vi "报告生成子VI.vi"(5 "column width (1)":dbl=10.0 format="%#_13g", 6 "error in (no error)":errorcluster caption="错误输入（无错误）", 7 "产品编号":string, 8 "text data":string[][](array[string]) caption="文本数据", 9 "报告保存路径":path, 10 "标注后的图片路径":path, 11 "报告模板路径":path) -> (2 "报告存储路径":path, 3 "标注后的图片存储路径":path)   [LabVIEW 2018]
uses:
  <vilib>/Utility/NIReport.llb/HTML Report Image Alignment.ctl
  <vilib>/Utility/NIReport.llb/Report Type.ctl
  <vilib>/Utility/NIReport.llb/Append Report Text (str wrap).vi
  <vilib>/Utility/NIReport.llb/Append Text Table to Report (wrap).vi
  <vilib>/Utility/NIReport.llb/Append Image to Report (path wrap).vi
  <vilib>/Utility/NIReport.llb/NI_report.lvclass
  <vilib>/Utility/NIReport.llb/Word/NI_Word.lvclass
  <vilib>/Utility/NIReport.llb/NI_ReportGenerationCore.lvlib
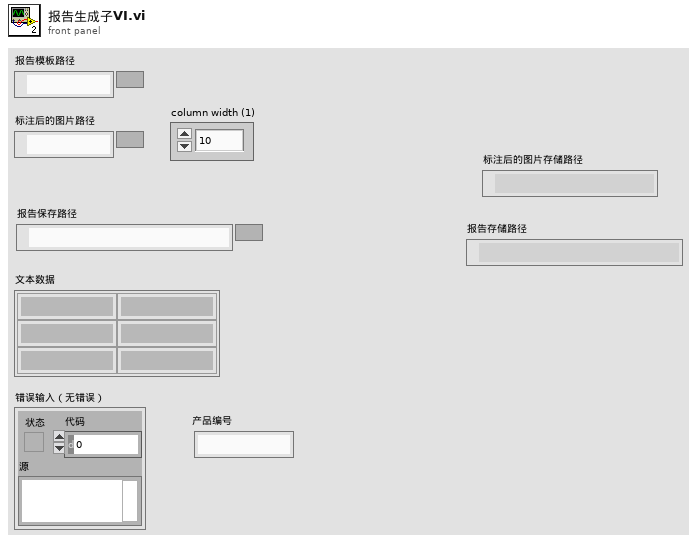
[diagram p1: front panel]
types:
  T1 = typedef "NI_ReportGenerationCore.lvlib/Report Type.ctl" = enum16{"HTML", "Word", "Excel"}
  T2 = cluster{"position (excel)":cluster{"row":i32, "column":i32}, "name (excel)":string, "bookmark (word)":string}
  T3 = typedef "NI_ReportGenerationCore.lvlib/HTML Report Image Alignment.ctl" = enum16{"(default)", "LEFT", "RIGHT", "TOP", "TEXTTOP", "MIDDLE", "ABSMIDDLE", "BASELINE", "BOTTOM", "ABSBOTTOM"}
  T4 = enum16{"maximized", "minimized", "normal", "no change"}
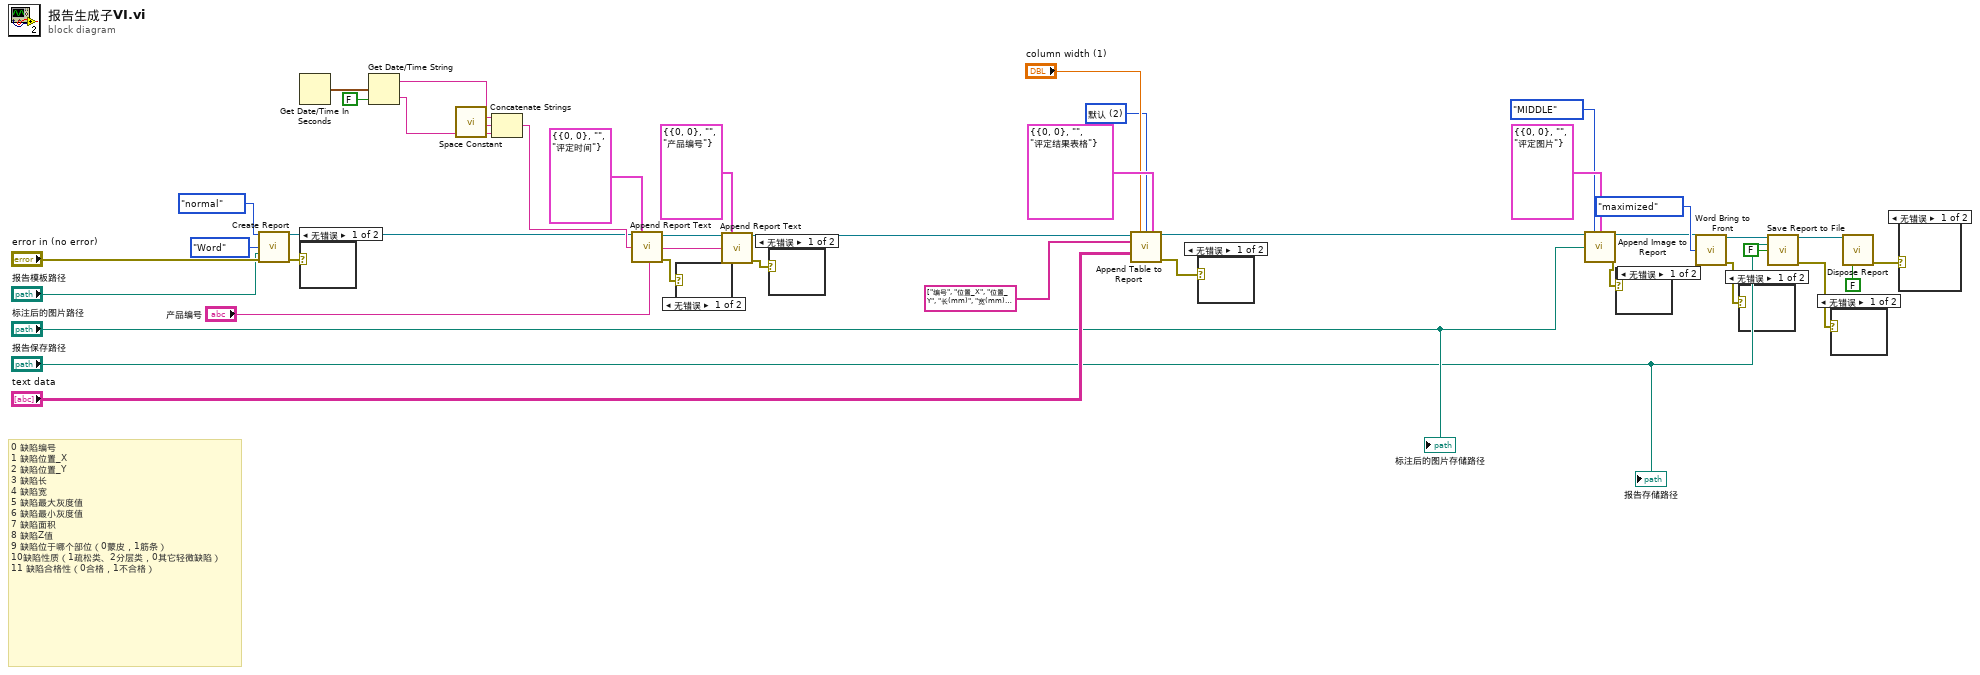
[diagram p0: block diagram]
diagram:
  w5 = u16 2 items=["US", "公制", "默认"] ("measurement system")
  # "0 缺陷编号\n1 缺陷位置_X\n2 缺陷位置_Y\n3 缺陷长\n4 缺陷宽\n5 缺陷最大灰度值\n6 缺陷最小灰度值\n7 缺陷面积\n8 缺陷Z值\n9 缺陷位于哪个部位（0蒙皮，1筋条）\n10缺陷性质（1疏松类、2分层类，0其它轻微缺陷）\n11 缺陷合格性（0合格，1不合格）"
  n1 = call <vilib>:"Create Report.vi"("window state (normal)"=T4."normal", "report type"=Report_Type."Word", "template (empty)"="报告模板路径", "error in (no error)"="error in (no error)") -> ("report out"=w1:refnum<class "NI_report.lvclass">, "error out"=w6:errorcluster)  [unwired: 10 in]
  n2 = Get Date/Time In Seconds() -> (seconds since 1Jan1904=w39:timestamp)
  n3 = case shown="无错误" w6 {
    frame No Error {
    }
    frame Error {
    }
  }
  n4 = Get Date/Time String(seconds (now)=w39, want seconds? (F)=FALSE ("需要秒？(F)")) -> (date string=w34:string, time string=w36:string)  [unwired: 1 in]
  n5 = call <vilib>:"Space Constant.vi"() -> ("String"=w33:string)
  n6 = Concatenate Strings(w34, w33, w36) -> (w35:string)
  n7 = call-poly <vilib>:"Append Report Text.vi"("report in"=w1, "MS Office parameters"=T2 {"position (excel)"={"row"=0, "column"=0}, "name (excel)"="", "bookmark (word)"="评定时间"}, "text"=w35) -> ("report out"=w26:refnum<class "NI_report.lvclass">, "error out"=w7:errorcluster)  [unwired: 9 in, 2 out]
  n8 = case shown="无错误" w7 {
    frame No Error {
    }
    frame Error {
    }
  }
  n9 = call-poly <vilib>:"Append Report Text.vi"("report in"=w26, "MS Office parameters"=T2 {"position (excel)"={"row"=0, "column"=0}, "name (excel)"="", "bookmark (word)"="产品编号"}, "text"="产品编号") -> ("report out"=w3:refnum<class "NI_report.lvclass">, "error out"=w4:errorcluster)  [unwired: 9 in, 2 out]
  n10 = case shown="无错误" w4 {
    frame No Error {
    }
    frame Error {
    }
  }
  n11 = call-poly <vilib>:"Append Table to Report.vi"("report in"=w3, "column width (1)"="column width (1)", "measurement system"=w5, "MS Office parameters"=T2 {"position (excel)"={"row"=0, "column"=0}, "name (excel)"="", "bookmark (word)"="评定结果表格"}, "column headers"=string[] ["编号", "位置_X", "位置_Y", "长(mm)", "宽(mm)", "最大灰度值", "最小灰度值", "面积(mm2)", "Z值(mm)", "部位", "类型", "合格性"], "text data"="text data") -> ("report out"=w2:refnum<class "NI_report.lvclass">, "error out"=w18:errorcluster)  [unwired: 6 in, 2 out]
  n12 = case shown="无错误" w18 {
    frame No Error {
    }
    frame Error {
    }
  }
  n13 = call-poly <vilib>:"Append Image to Report.vi"("report in"=w2, "alignment (default)"=HTML_Report_Image_Alignment."MIDDLE", "MS Office parameters"=T2 {"position (excel)"={"row"=0, "column"=0}, "name (excel)"="", "bookmark (word)"="评定图片"}, "path or URL of image"="标注后的图片路径") -> ("report out"=w28:refnum<class "NI_report.lvclass">, "error out"=w10:errorcluster)  [unwired: 8 in, 2 out]
  n14 = case shown="无错误" w10 {
    frame No Error {
    }
    frame Error {
    }
  }
  n15 = call <vilib>:"Word Bring to Front.vi"("report in"=w28, "window state (maximized)"=enum16{"maximized", "minimized", "normal"}."maximized") -> ("report out"=w29:refnum<class "NI_report.lvclass">, "error out"=w8:errorcluster)  [unwired: 12 in]
  n16 = case shown="无错误" w8 {
    frame No Error {
    }
    frame Error {
    }
  }
  n17 = call-dynamic "Save Report to File.vi"("report in"=w29, "report file path"="报告保存路径", "prompt to replace? (F)"=FALSE) -> ("report out"=w17:refnum<class "NI_report.lvclass">, "error out"=w9:errorcluster)  [unwired: 11 in]
  n18 = case shown="无错误" w9 {
    frame No Error {
    }
    frame Error {
    }
  }
  n19 = call-dynamic "Dispose Report.vi"("report in"=w17, "close report? (T)"=FALSE ("save changes? (F)")) -> ("error out"=w19:errorcluster)  [unwired: 13 in]
  n20 = case shown="无错误" w19 {
    frame No Error {
    }
    frame Error {
    }
  }
  "标注后的图片存储路径" <- "标注后的图片路径"
  "报告存储路径" <- "报告保存路径"
